vi "set_ref_clus_THCD_400.vi"(6 "variable_ref":T1, 8 "FM1":dbl, 9 "FC2":dbl, 10 "FC1":dbl, 11 "status":bool) -> ()   [LabVIEW 2019]
uses:
  thcd_controls/variable_reference.ctl
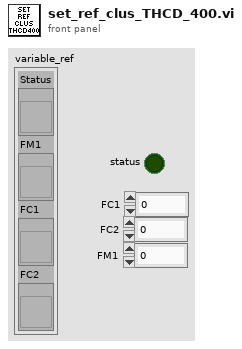
[diagram p1: front panel]
types:
  T1 = typedef "variable_reference.ctl" = cluster{"Status":refnum<vi>, "FM1":refnum<vi>, "FC1":refnum<vi>, "FC2":refnum<vi>}
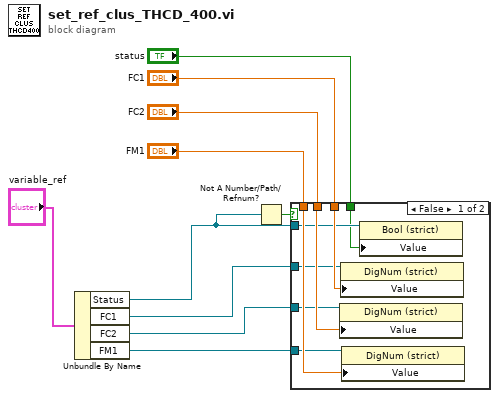
[diagram p0: block diagram]
diagram:
  n1 = Unbundle By Name("variable_ref") -> ("Status"=w6:refnum<vi>, "FC1"=w7:refnum<vi>, "FC2"=w8:refnum<vi>, "FM1"=w9:refnum<vi>)
  n2 = Not A Number/Path/Refnum?(number/path/refnum=w6) -> (NaN/Path/Refnum?=w10:bool)
  n3 = case shown="False" w10 {
    tunnel: "FC1" -> [w18 _]
    tunnel: "FC2" -> [w17 _]
    tunnel: "FM1" -> [w16 _]
    tunnel: w7 -> [w15 _]
    tunnel: w8 -> [w14 _]
    tunnel: w9 -> [w13 _]
    tunnel: w6 -> [w12 _]
    tunnel: "status" -> [w11 _]
    frame False {
      n4 = property class="DigNum (strict)"(reference=w14, "Value"=w17) -> ()  [unwired: 1 in, 2 out]
      n5 = property class="DigNum (strict)"(reference=w15, "Value"=w18) -> ()  [unwired: 1 in, 2 out]
      n6 = property class="DigNum (strict)"(reference=w13, "Value"=w16) -> ()  [unwired: 1 in, 2 out]
      n7 = property class="Bool (strict)"(reference=w12, "Value"=w11) -> ()  [unwired: 1 in, 2 out]
    }
    frame True {
    }
  }
